vi "getNewValueXML.vi"(8 "error in (no error)":errorcluster, 11 "RfRamp in":refnum<class "RfRamp.lvclass">) -> (0 "error out":errorcluster, 2 "newValueXML":refnum<class "xmlNode.lvclass">, 3 "RfRamp out":refnum<class "RfRamp.lvclass">)   [LabVIEW 2009, in "Tools.lvlib" / "Scripting.lvlib" / "RfRamp.lvclass"]
uses:
  RfRamp.lvclass
  xmlNode/xmlNode.lvclass
  RfRamp.lvclass/RfRamp.ctl
  ScriptEvent.lvclass
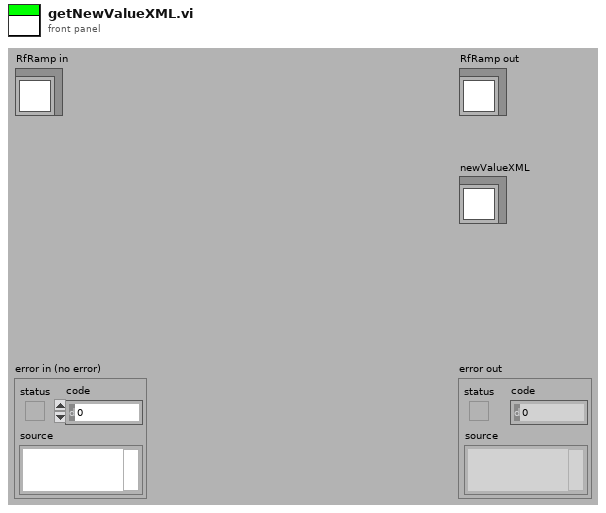
[diagram p1: front panel]
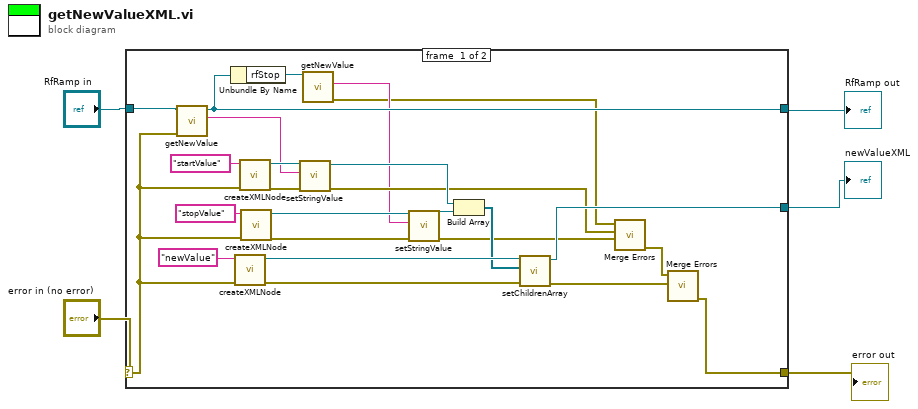
[diagram p0: block diagram]
diagram:
  n1 = case shown="No Error" "error in (no error)" {
    selector: "error in (no error)" -> [w26 w32]
    tunnel: [w10 w32] -> w3
    tunnel: [w8 w31] -> w4
    tunnel: "RfRamp in" -> [w29 w31]
    tunnel: [w18 _] -> w2
    frame #0 {
      n2 = call "getNewValue.vi"("error in (no error)"=w26, "ScriptEvent.lvclass in"=w29) -> ("newValue"=w23:string, "ScriptEvent.lvclass out"=w8:refnum<class "RfRamp.lvclass">)  [unwired: 7 in, 1 out]
      n3 = Unbundle By Name(w8) -> ("rfStop"=w9:refnum<class "rf.lvclass">)
      n4 = call "createXMLNode.vi"("error in (no error)"=w26, "name"="newValue") -> ("error out"=w19:errorcluster, "xmlNode out"=w20:refnum<class "xmlNode.lvclass">)  [unwired: 8 in]
      n5 = call "createXMLNode.vi"("error in (no error)"=w26, "name"="startValue") -> ("error out"=w24:errorcluster, "xmlNode out"=w25:refnum<class "xmlNode.lvclass">)  [unwired: 8 in]
      n6 = call "createXMLNode.vi"("error in (no error)"=w26, "name"="stopValue") -> ("error out"=w21:errorcluster, "xmlNode out"=w22:refnum<class "xmlNode.lvclass">)  [unwired: 8 in]
      n7 = call-dynamic "setStringValue.vi"("error in (no error)"=w24, "stringValue"=w23, "xmlNode.lvclass in"=w25) -> ("error out"=w14:errorcluster, "xmlNode.lvclass out"=w17:refnum<class "xmlNode.lvclass">)  [unwired: 7 in]
      n8 = call "getNewValue.vi"("ScriptEvent.lvclass in"=w9) -> ("error out"=w6:errorcluster, "newValue"=w7:string)  [unwired: 8 in, 1 out]
      n9 = call-dynamic "setStringValue.vi"("error in (no error)"=w21, "stringValue"=w7, "xmlNode.lvclass in"=w22) -> ("error out"=w13:errorcluster, "xmlNode.lvclass out"=w16:refnum<class "xmlNode.lvclass">)  [unwired: 7 in]
      n10 = Build Array(w17, w16) -> (w15:refnum<class "xmlNode.lvclass">[])
      n11 = call-dynamic "setChildrenArray.vi"("error in (no error)"=w19, "Children"=w15, "xmlNode.lvclass in"=w20) -> ("error out"=w11:errorcluster, "xmlNode.lvclass out"=w18:refnum<class "xmlNode.lvclass">)  [unwired: 7 in]
      n12 = call <vilib>:"Merge Errors.vi"("error in 3 (no error)"=w13, "error in 2 (no error)"=w14, "error in 1 (no error)"=w6) -> ("error out"=w12:errorcluster)  [unwired: 4 in]
      n13 = call <vilib>:"Merge Errors.vi"("error in 2 (no error)"=w11, "error in 1 (no error)"=w12) -> ("error out"=w10:errorcluster)  [unwired: 5 in]
    }
    frame #1 {
    }
  }
  "error out" <- w3
  "RfRamp out" <- w4
  "newValueXML" <- w2
